vi "multiply.vi"() -> ()   [LabVIEW 2011]
panel:
  out "x*y":dbl
  in  "Numeric 2":dbl
  in  "Numeric":dbl
  in  "stop":bool
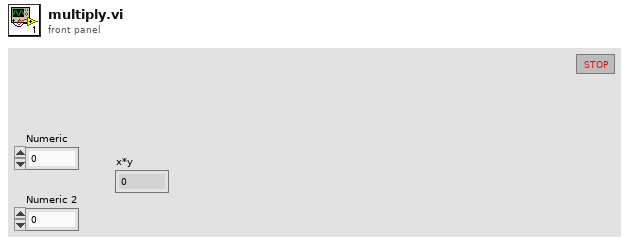
[diagram p1: front panel]
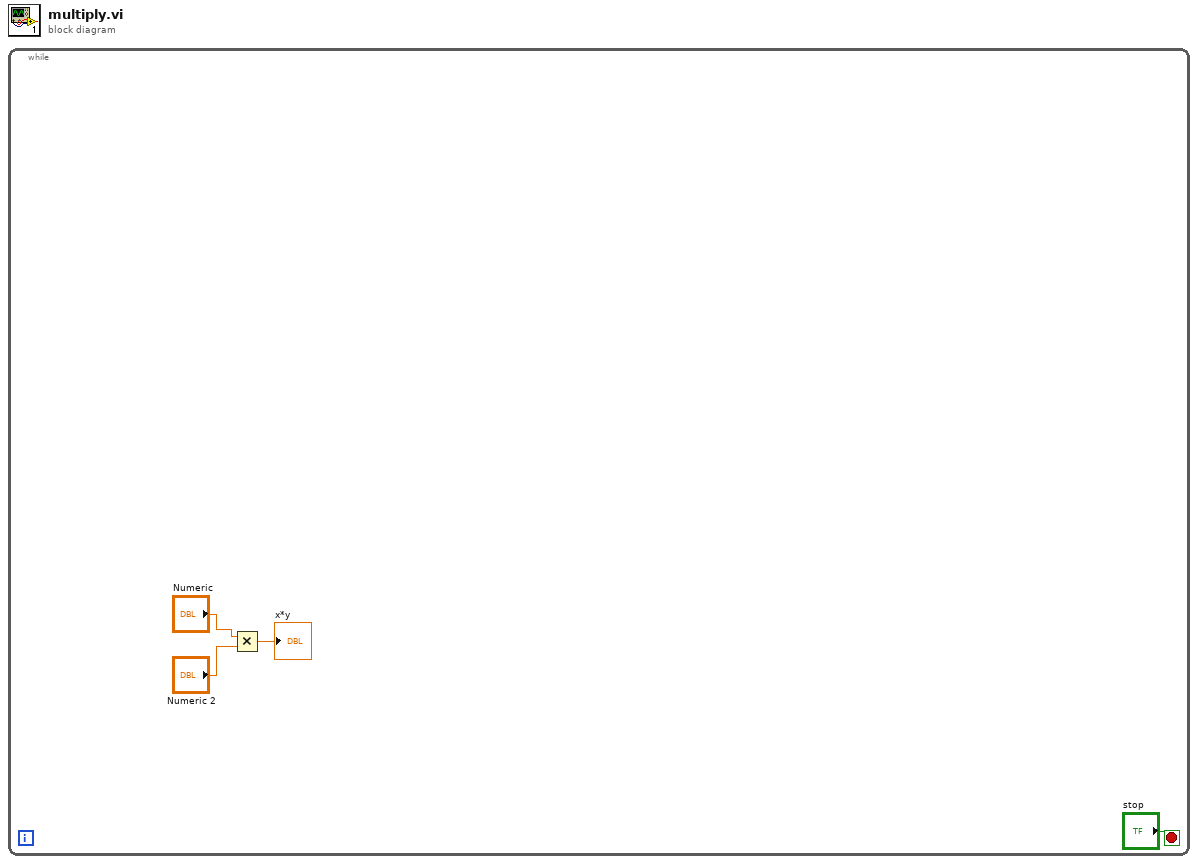
[diagram p0: block diagram]
diagram:
  n1 = while {
    stop <- "stop" stop-if-true
    n2 = Multiply(x="Numeric", y="Numeric 2") -> (x*y=→"x*y":dbl)
  }
